vi "Side Angle Calculation.vi"(11 "Diamond Targets":T1[](array[typedef])) -> (3 "Target Angle":dbl)   [LabVIEW 2011]
uses:
  Diamond Target Output.ctl
  Rectangle Position.ctl
  Target Confidence.ctl
panel:
  out "acos":dbl
  out "Right Theta":dbl
  out "Left Theta":dbl
  # "Side Angle was supposed to use the left/right targets to compute side angle, but we never finished it"
  # "I would not expect it to work at all"
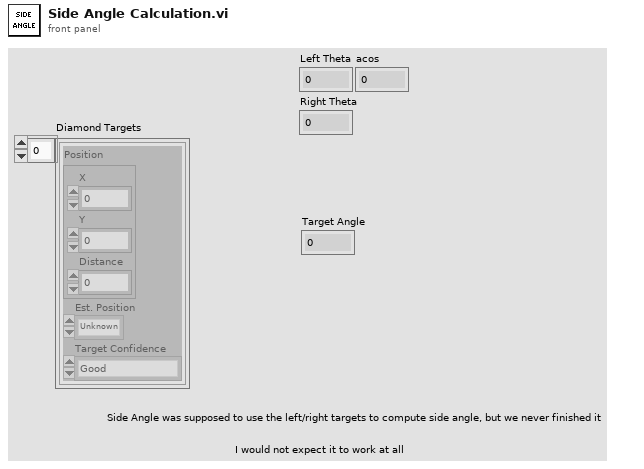
[diagram p1: front panel]
types:
  T1 = typedef "Diamond Target Output.ctl" = cluster{"Position":cluster{"X":dbl, "Y":dbl, "Distance":dbl}, "Est. Position":T2, "Target Confidence":T3}
  T2 = typedef "Rectangle Position.ctl" = enum16{"Unknown", "Top", "Right", "Left", "Bottom"}
  T3 = typedef "Target Confidence.ctl" = enum16{"Good", "Good-Clipped Y", "Marginal-Clipped X"}
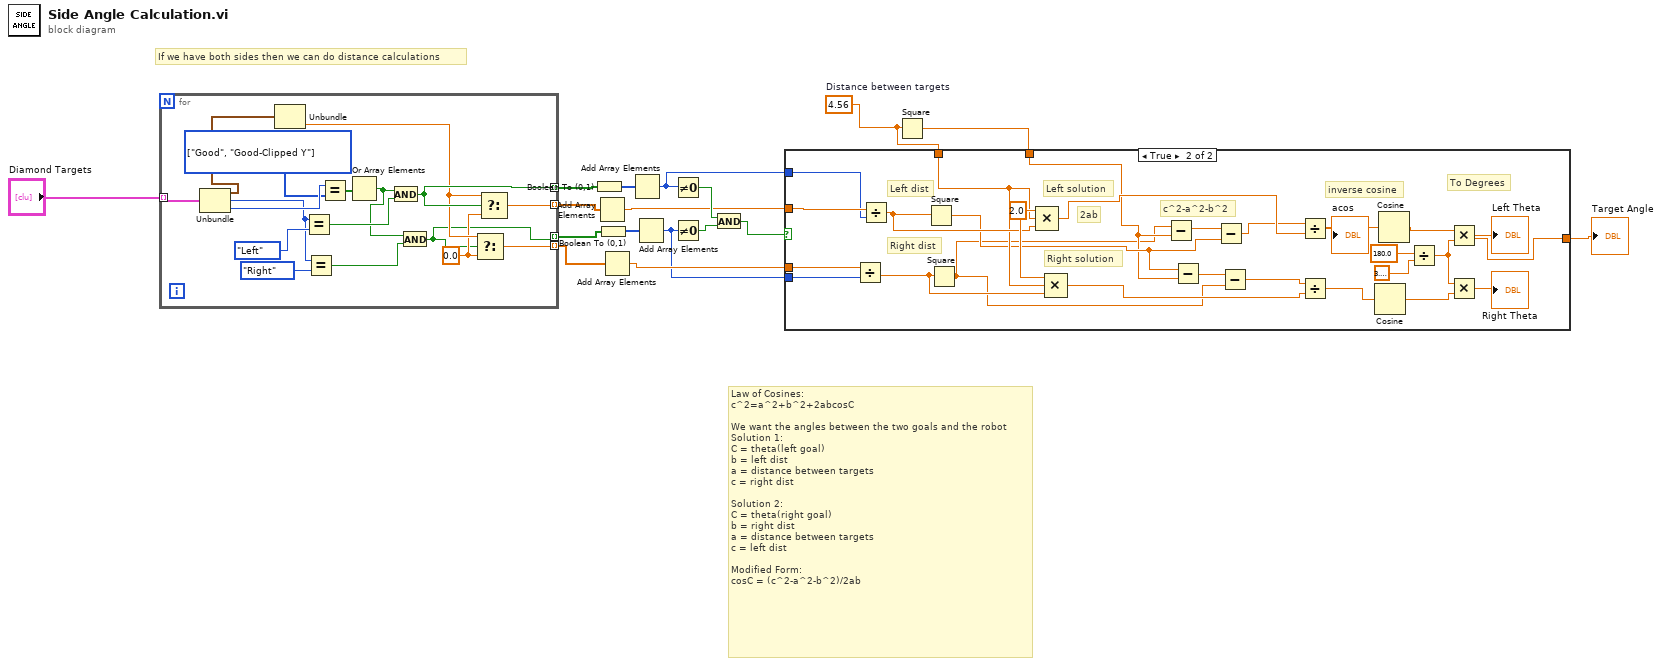
[diagram p0: block diagram]
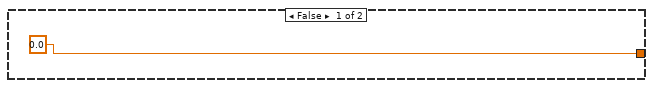
[diagram p2: hidden frame]
diagram:
  w1 = 4.56  # Distance between targets
  # "Law of Cosines:\nc^2=a^2+b^2+2abcosC\n\nWe want the angles between the two goals and the robot\nSolution 1: \nC = theta(left goal)\nb = left dist\na = distance between targets\nc = right dist\n\nSolution 2:\nC = theta(right goal)\nb = right dist\na = distance between targets\nc = left dist\n\nModified Form:\ncosC = (c^2-a^2-b^2)/2ab"
  # "If we have both sides then we can do distance calculations"
  n1 = for {
    tunnel: "Diamond Targets" -> [w34] mode=indexing
    tunnel: [w23] -> w8 mode=indexing
    tunnel: [w22] -> w16 mode=indexing
    tunnel: [w19] -> w5 mode=indexing
    tunnel: [w18] -> w15 mode=indexing
    w20 = 0.0 ("f")
    w32 = T3[] [enum."Good", enum."Good-Clipped Y"] items=["Good", "Good-Clipped Y", "Marginal-Clipped X"]
    n2 = Unbundle(w34) -> ("Position"=w24:cluster{"X":dbl, "Y":dbl, "Distance":dbl}, "Est. Position"=w30:T2, "Target Confidence"=w33:T3)
    n3 = Unbundle(w24) -> ("Distance"=w21:dbl)  [unwired: 2 out]
    n4 = Equal?(x=w30, y=Rectangle_Position."Left") -> (x = y?=w28:bool)
    n5 = Equal?(x=w30, y=Rectangle_Position."Right") -> (x = y?=w27:bool)
    n6 = Equal?(x=w33, y=w32) -> (x = y?=w26:bool[])
    n7 = Or Array Elements(Boolean array=w26) -> (logical OR=w25:bool)
    n8 = And(x=w25, y=w28) -> (x .and. y?=w22:bool)
    n9 = And(x=w25, y=w27) -> (x .and. y?=w18:bool)
    n10 = Select(t=w21, s=w18, f=w20) -> (s? t:f=w19:dbl)
    n11 = Select(t=w21, s=w22, f=w20) -> (s? t:f=w23:dbl)
  }
  n12 = Boolean To (0,1)(Boolean=w16) -> (0, 1=w14:i16[])
  n13 = Add Array Elements(numeric array=w8) -> (sum=w7:dbl)
  n14 = Boolean To (0,1)(Boolean=w15) -> (0, 1=w13:i16[])
  n15 = Add Array Elements(numeric array=w5) -> (sum=w4:dbl)
  n16 = Add Array Elements(numeric array=w14) -> (sum=w6:i16)
  n17 = Add Array Elements(numeric array=w13) -> (sum=w3:i16)
  n18 = Not Equal To 0?(x=w6) -> (x != 0?=w12:bool)
  n19 = Not Equal To 0?(x=w3) -> (x != 0?=w11:bool)
  n20 = And(x=w12, y=w11) -> (x .and. y?=w10:bool)
  n21 = Square(x=w1) -> (x^2=w2:dbl)
  n22 = case shown="True" w10 {
    tunnel: [0.0 w45] -> w9
    tunnel: w7 -> [_ w61]
    tunnel: w6 -> [_ w60]
    tunnel: w4 -> [_ w59]
    tunnel: w3 -> [_ w58]
    tunnel: w2 -> [_ w41]
    tunnel: w1 -> [_ w54]
    frame False {
    }
    frame True {
      w57 = 2.0 ("value")
      # "To Degrees"
      # "inverse cosine"
      # "c^2-a^2-b^2"
      # "2ab"
      # "Right solution"
      # "Left solution"
      # "Right dist"
      # "Left dist"
      n23 = Divide(x=w59, y=w58) -> (x/y=w55:dbl)
      n24 = Divide(x=w61, y=w60) -> (x/y=w56:dbl)
      n25 = Square(x=w56) -> (x^2=w42:dbl)
      n26 = Square(x=w55) -> (x^2=w39:dbl)
      n27 = Compound Arithmetic op=MULTIPLY(w57, w54, w56) -> (w53:dbl)
      n28 = Compound Arithmetic op=MULTIPLY(w57, w54, w55) -> (w52:dbl)
      n29 = Subtract(x=w39, y=w41) -> (x-y=w44:dbl)
      n30 = Subtract(x=w42, y=w41) -> (x-y=w40:dbl)
      n31 = Subtract(x=w44, y=w42) -> (x-y=w43:dbl)
      n32 = Subtract(x=w40, y=w39) -> (x-y=w38:dbl)
      n33 = Divide(x=w43, y=w53) -> (x/y=w36:dbl)
      "acos" <- w36
      n34 = Divide(x=w38, y=w52) -> (x/y=w51:dbl)
      n35 = Cosine(x=w51) -> (cos(x)=w48:dbl)
      n36 = Cosine(x=w36) -> (cos(x)=w37:dbl)
      n37 = Divide(x=180.0, y=3.141592653589793) -> (x/y=w49:dbl)
      n38 = Multiply(x=w37, y=w49) -> (x*y=w45:dbl)
      "Left Theta" <- w45
      n39 = Multiply(x=w49, y=w48) -> (x*y=→"Right Theta":dbl)
    }
  }
  "Target Angle" <- w9
